vi "Read IPG Thermistor Temperature.vi"(8 "error in":errorcluster, 9 "Abort Threshold (42 C)":dbl=42.0 format="%5.5f", 10 "Critical Threshold (41 C)":dbl=41.0 format="%5.5f", 11 "Warning Threshold (40 C)":dbl=40.0 format="%5.5f") -> (0 "error out":errorcluster, 1 "Data":string, 2 "Response Token":string, 3 "Compensated Temperature (C)":dbl=nan)   [LabVIEW 2010]
doc: "This function gets the xPG internal temperature. If GEN CAL parameters are provided, then the temperature value will be compensated."
uses:
  Typedef Command List.ctl
panel:
  # "GEN CALS"
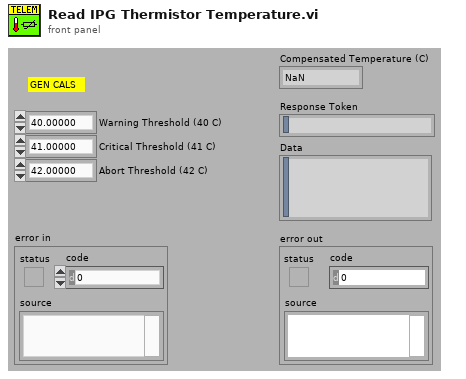
[diagram p1: front panel]
types:
  T1 = typedef "Typedef Command List.ctl" = enum16{"Get xPG Status", "xPG Stimulation", "Select Program", "Increment Program Amplitude", "Decrement Program Amplitude", "Get PoP Constants", "Get PPC Constants", "Get Program Names", "Set Pulse Amplitude", "Increment Pulse Amplitude", "Decrement Pulse Amplitude", "Get Pulse Widths", "Set Pulse Widths", "Increment Pulse Width", "Decrement Pulse Width", "Get Program Frequency", "Set Program Frequency", "Increment Program Frequency", "Decrement Program Frequency", "Inject Event", "Charging Control", "Get xPG Identity", "Set xPG Identity", "Restore Program Defaults", "Get Program Definition", "Set Program Definition", "Get Program Constants", "Set Program Constants", "Get Configurable Device Parameters", "Set Configurable Device Parameters", "Get Pulse Constants", "Set Pulse Constants", "Get Lead Limits", "Set Lead Limits", "Get Channel Calibrations", "Set Channel Calibrations", "<reserved 2>", "<reserved 3>", "<reserved 4>", "<reserved 5>", "<reserved 6>", "<reserved 7>", "Get Stim Asic HV Calibrations", "Set Stim Asic HV Calibrations", "<reserved 8>", "<reserved 9>", "Get CP Data", "Set CP Data", "Clear Log", "Read Log", "Append Log", "Get Patient Program Runtime", "Set Patient Program Runtime", "Impedance Measurement", "Enter Storage Mode", "Echo Short", "Echo Long", "Get General Calibration", "Set General Calibration", "Get Trim List", "Set Trim List", "Get Counter", "Set Counter", "Get Test Stimulation", "Set Test Stimulation", "Get Titration Stimulation", "Set Titration Stimulation", "Get Ramp Time", "Set Ramp Time", "Get VBAT", "Set Software Description Block", "Get Software Description Block", "Write Memory", "Read Memory", "Reset xPG", "Erase Flash Block", "Write Vectors", "Read Vectors", "Diagnostic Data", "Set Background Impedance", "Get Background Impedence ", "Set Test Waveform", "Calibrate Channel", "Get Log Range", "Reserved 0x55", "Reserved 0x56", "MICS Options", "Pair PPC", "Pair POP", "Stop Bootloader", "Tune MICS", "MICS Diagnostics", "Undefined"}
  T2 = cluster{"Command":T1, "Function":enum16{"Open Session", "Close Session", "Downlink Only", "Uplink Only", "Transceive (DN -> UP)"}, "MICS_ID":u32, "EXID":u32, "Use Local":bool, "Transceive Delay mS":dbl, "CP_DATA IN":u8[], "Parameters":string}
  T3 = enum16{"Open Session", "Close Session", "Downlink Only", "Uplink Only", "Transceive (DN -> UP)"}
  T4 = cluster{"Response Token":string, "Response Code":string, "bChecksum Valid":bool, "tChecksum Valid":bool, "CP_DATA OUT":u8[], "Data":string}
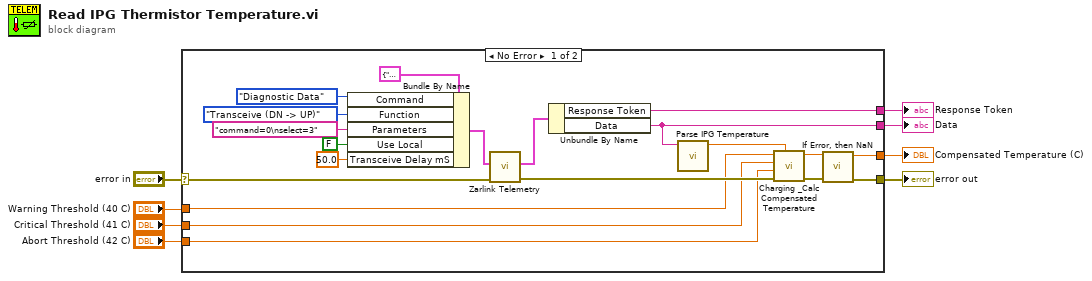
[diagram p0: block diagram]
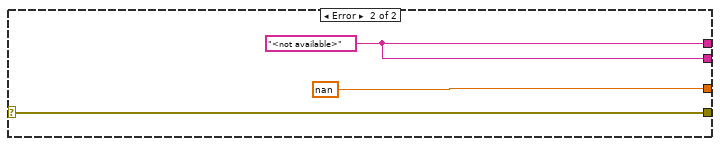
[diagram p2: hidden frame]
diagram:
  n1 = case shown="No Error" "error in" {
    selector: "error in" -> [w15 w31]
    tunnel: [w21 w31] -> w7
    tunnel: [w20 nan ("Temperature")] -> w6
    tunnel: [w19 w29] -> w5
    tunnel: [w18 w29] -> w4
    tunnel: "Warning Threshold (40 C)" -> [w14 _]
    tunnel: "Critical Threshold (41 C)" -> [w11 _]
    tunnel: "Abort Threshold (42 C)" -> [w10 _]
    frame No Error {
      n2 = Bundle By Name(cluster=T2 {"Command"=enum."Get xPG Status", "Function"=enum."Close Session", "MICS_ID"=0, "EXID"=16773121, "Use Local"=FALSE, "Transceive Delay mS"=100.0, "CP_DATA IN"=[], "Parameters"=""} ("Input"), "Command"=Typedef_Command_List."Diagnostic Data", "Function"=T3."Transceive (DN -> UP)", "Parameters"="command=0\nselect=3", "Use Local"=FALSE, "Transceive Delay mS"=50.0) -> (w28:T2)
      n3 = call "Zarlink Telemetry.vi"("error in (no error)"=w15, "Input"=w28) -> ("error out"=w17:errorcluster, "Output"=w22:T4)  [unwired: 7 in, 1 out]
      n4 = Unbundle By Name(w22) -> ("Response Token"=w18:string, "Data"=w19:string)
      n5 = call "Parse IPG Temperature.vi"("Thermistor Data"=w19) -> ("Temperature C"=w13:dbl)  [unwired: 9 in, 1 out]
      n6 = call "Charging _Calc Compensated Temperature.vi"("target temperature (C)"=w13, "error in"=w17, "Abort Threshold (42 C)"=w10, "Critical Threshold (41 C)"=w11, "Warning Threshold (40 C)"=w14) -> ("error out"=w16:errorcluster, "compensated temperature (C)"=w12:dbl)  [unwired: 2 in, 1 out]
      n7 = call "If Error, then NaN.vi"("error in (T)"=w16, "value1"=w12) -> ("error out"=w21:errorcluster, "value out1"=w20:dbl)  [unwired: 4 in, 2 out]
    }
    frame Error {
      w29 = "<not available>" ("Response Token")
    }
  }
  "error out" <- w7
  "Compensated Temperature (C)" <- w6
  "Data" <- w5
  "Response Token" <- w4
